vi "find and set output refs.vi"(8 "error in (no error)":errorcluster, 10 "Device Info in":T2 {"Outputs"."Output References"."Holding Registers" format="%.0x"; "Outputs"."Output References"."Coils" format="%.0x"; "Inputs"."Input References"."Input Registers" format="%.0x"; "Inputs"."Input References"."Discrete Inputs" format="%.0x"; "Interface Data"."Serial Settings"."parity (even)" items=["None", "Odd", "Even", "Mark", "Space"]; "Interface Data"."Serial Settings"."flow control (none)" items=["None", "XON/XOFF", "RTS/CTS", "XON/XOFF & RTS/CTS", "DTR/DSR", "XON/XOFF & DTR/DSR"]}, 11 "Device Reference in":T1 format="%.0x") -> (0 "error out":errorcluster, 2 "Device Info out":T2 {"Outputs"."Output References"."Holding Registers" format="%.0x"; "Outputs"."Output References"."Coils" format="%.0x"; "Inputs"."Input References"."Input Registers" format="%.0x"; "Inputs"."Input References"."Discrete Inputs" format="%.0x"; "Interface Data"."Serial Settings"."parity (even)" items=["None", "Odd", "Even", "Mark", "Space"]; "Interface Data"."Serial Settings"."flow control (none)" items=["None", "XON/XOFF", "RTS/CTS", "XON/XOFF & RTS/CTS", "DTR/DSR", "XON/XOFF & DTR/DSR"]}, 3 "Device Ref out":T1 format="%.0x")   [LabVIEW 2015]
uses:
  Shared/Device Info.ctl
  Shared/Controls/Interface Type.ctl
  Shared/Controls/Data Model/TCP Settings.ctl
  Shared/Controls/Data Model/Serial Settings.ctl
  Shared/Controls/Data Model/Inputs.ctl
  Shared/Controls/Data Model/Input Channel Data.ctl
  Shared/Controls/Data Model/Channel.ctl
  System Explorer/SubVIs/Modbus Type.ctl
  Shared/Controls/Data Model/Mapping.ctl
  Shared/Controls/Data Model/DataType.ctl
  Shared/Controls/Data Model/Input References.ctl
  <vilib>/NI Veristand/Custom Device API/Custom Device Item Ref.ctl
  Shared/Controls/Data Model/Outputs.ctl
  Shared/Controls/Data Model/Output Channel Data.ctl
  Shared/Controls/Data Model/Output References.ctl
  <vilib>/NI Veristand/Custom Device API/Custom Device Channel Type.ctl
  Shared/Constants.vi
  <vilib>/NI VeriStand/Custom Device API/Custom Device API.lvlib
  Shared/Modbus Master Shared.lvlib
  System Explorer/Modbus Master System Explorer.lvlib
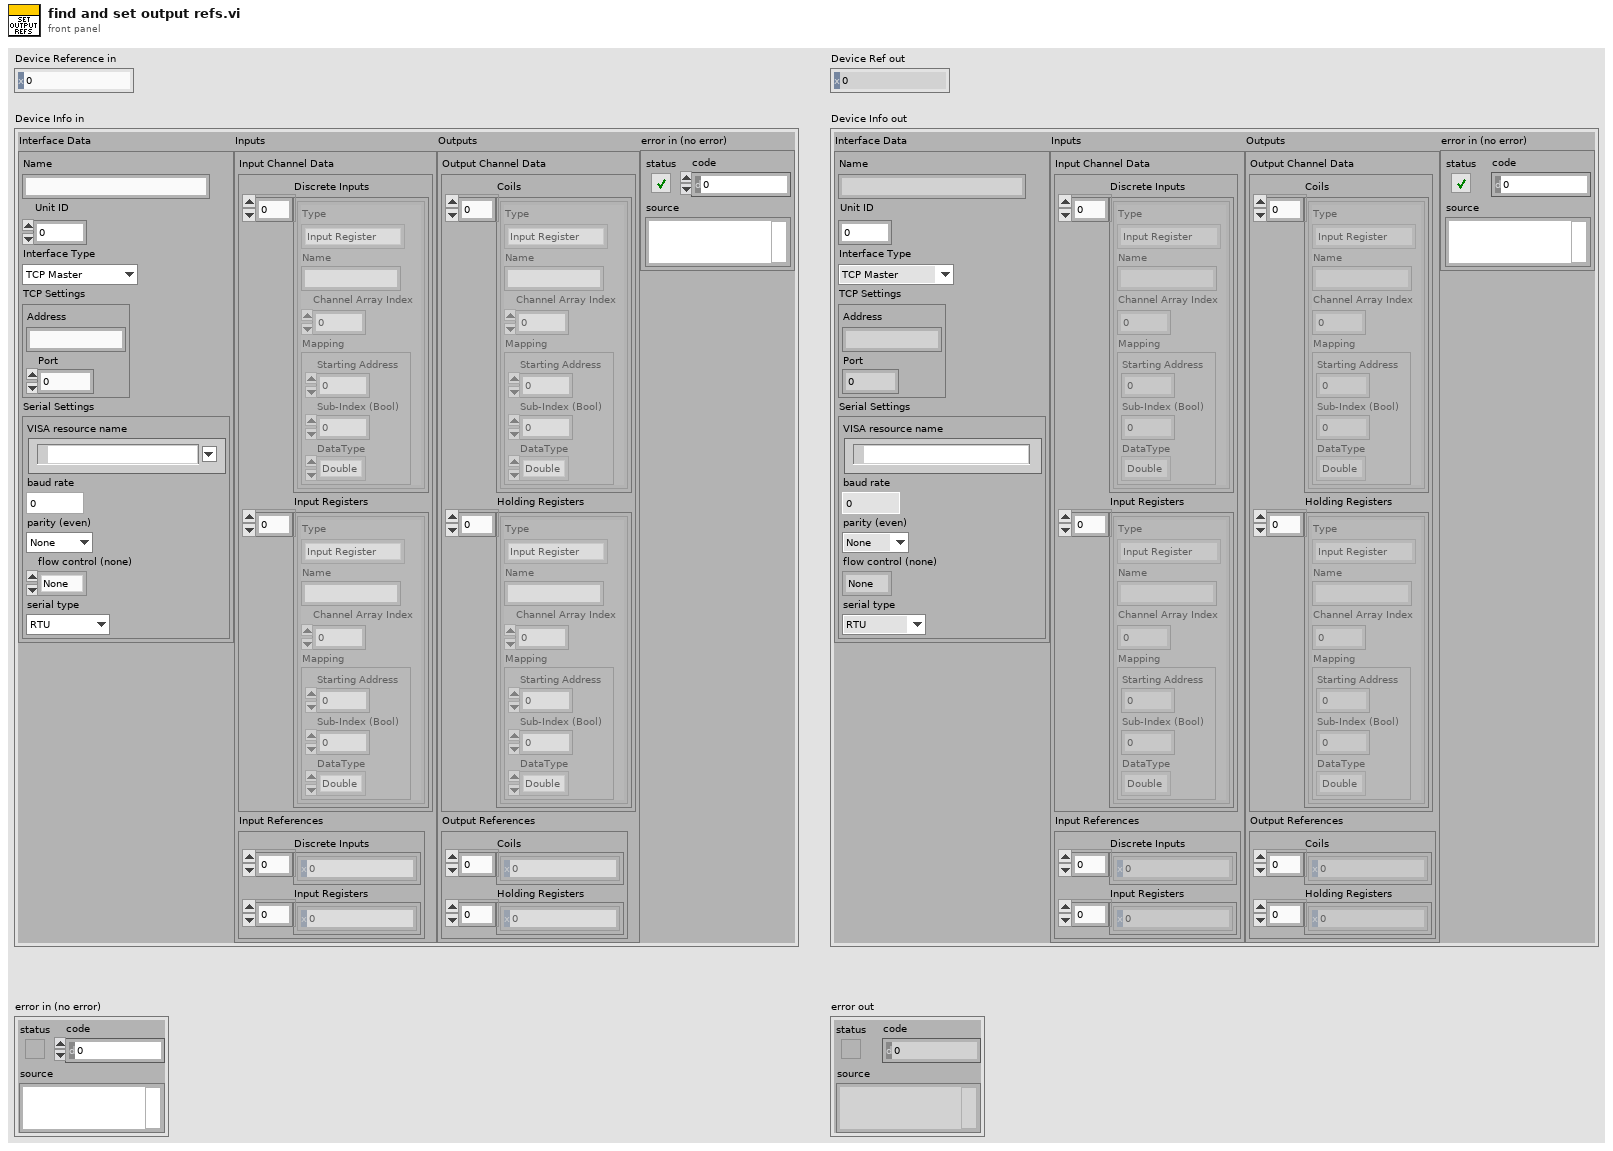
[diagram p1: front panel]
types:
  T1 = typedef "Custom Device API.lvlib/Custom Device Item Ref.ctl" = u64
  T2 = typedef "Modbus Master Shared.lvlib/Device Info.ctl" = cluster{"Interface Data":cluster{"Name":string, "Unit ID":u8, "Interface Type":T3, "TCP Settings":T4, "Serial Settings":T5}, "Inputs":T6, "Outputs":T13, "error in (no error)":errorcluster}
  T3 = typedef "Modbus Master System Explorer.lvlib/Interface Type.ctl" = enum16{"TCP Master", "Serial Master"}
  T4 = typedef "Modbus Master Shared.lvlib/TCP Settings.ctl" = cluster{"Address":string, "Port":u16}
  T5 = typedef "Modbus Master Shared.lvlib/Serial Settings.ctl" = cluster{"VISA resource name":refnum<visa-resource-name>, "baud rate":u32, "parity (even)":u16, "flow control (none)":u16, "serial type":enum16{"RTU", "ASCII"}}
  T6 = typedef "Modbus Master Shared.lvlib/Inputs.ctl" = cluster{"Input Channel Data":T7, "Input References":T12}
  T7 = typedef "Modbus Master Shared.lvlib/Input Channel Data.ctl" = cluster{"Discrete Inputs":T8[], "Input Registers":T8[]}
  T8 = typedef "Modbus Master Shared.lvlib/Channel.ctl" = cluster{"Type":T9, "Name":string, "Channel Array Index":i32, "Mapping":T10}
  T9 = typedef "Modbus Master Shared.lvlib/Modbus Type.ctl" = enum16{"Coil", "Discrete Input", "Holding Register", "Input Register"}
  T10 = typedef "Modbus Master Shared.lvlib/Mapping.ctl" = cluster{"Starting Address":u16, "Sub-Index (Bool)":u16, "DataType":T11}
  T11 = typedef "Modbus Master Shared.lvlib/DataType.ctl" = enum16{"Double", "Single", "I64", "I32", "I16", "I8", "U64", "U32", "U16", "U8", "Boolean", "String"}
  T12 = typedef "Modbus Master Shared.lvlib/Input References.ctl" = cluster{"Discrete Inputs":T1[], "Input Registers":T1[]}
  T13 = typedef "Modbus Master Shared.lvlib/Outputs.ctl" = cluster{"Output Channel Data":T14, "Output References":T15}
  T14 = typedef "Modbus Master Shared.lvlib/Output Channel Data.ctl" = cluster{"Coils":T8[], "Holding Registers":T8[]}
  T15 = typedef "Modbus Master Shared.lvlib/Output References.ctl" = cluster{"Coils":T1[], "Holding Registers":T1[]}
  T16 = typedef "Custom Device API.lvlib/Custom Device Channel Type.ctl" = enum16{"Input", "Output"}
  T17 = typedef "Custom Device API.lvlib/Custom Device Item Info.ctl" = cluster{"Name":string, "Is Channel":bool, "GUID":string, "Is Waveform":bool}
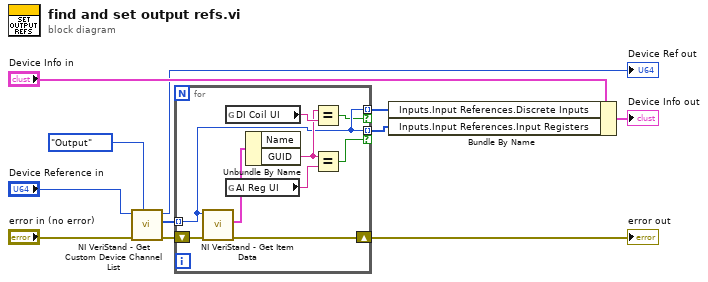
[diagram p0: block diagram]
diagram:
  n1 = call <vilib>:"NI VeriStand - Get Custom Device Channel List.vi"("Channel Type"=Custom_Device_Channel_Type."Output", "error in (no error)"="error in (no error)", "Device Ref in"="Device Reference in") -> ("error out"=w2:errorcluster, "Specified Channel Ref List"=w7:T1[], "Device Ref out"=→"Device Ref out":T1)  [unwired: 6 in]
  n2 = for {
    tunnel: w7 -> [w16] mode=indexing
    tunnel: [w16] -> w10 mode=indexing if=w15
    tunnel: [w16] -> w9 mode=indexing if=w14
    shift-right: [w12] -> w1
    shift-left: w2 -> [w13]
    n3 = call <vilib>:"NI VeriStand - Get Item Data.vi"("error in (no error)"=w13, "Item Ref in"=w16) -> ("error out"=w12:errorcluster, "Item Info"=w20:T17)  [unwired: 6 in, 2 out]
    n4 = global read "Constants.vi" "DI Coil UI"() -> (w18:string)
    n5 = global read "Constants.vi" "AI Reg UI"() -> (w19:string)
    n6 = Unbundle By Name(w20) -> ("GUID"=w17:string)  [unwired: 1 out]
    n7 = Equal?(x=w17, y=w18) -> (x = y?=w14:bool)
    n8 = Equal?(x=w17, y=w19) -> (x = y?=w15:bool)
  }
  "error out" <- w1
  n9 = Bundle By Name(cluster="Device Info in", "Inputs.Input References.Discrete Inputs"=w9, "Inputs.Input References.Input Registers"=w10) -> (→"Device Info out":T2)
